vi "Re-write README files.vi"() -> ()   [LabVIEW 2010]
uses:
  <vilib>/Utility/file.llb/Read From Spreadsheet File (string).vi
  <vilib>/Utility/file.llb/Write To Spreadsheet File (string).vi
panel:
  in  "System Save Button":bool
  in  "Primary Path":path
  out "Selected Paths":path[](array[path])
  in  "Readme Files":i32(listbox)
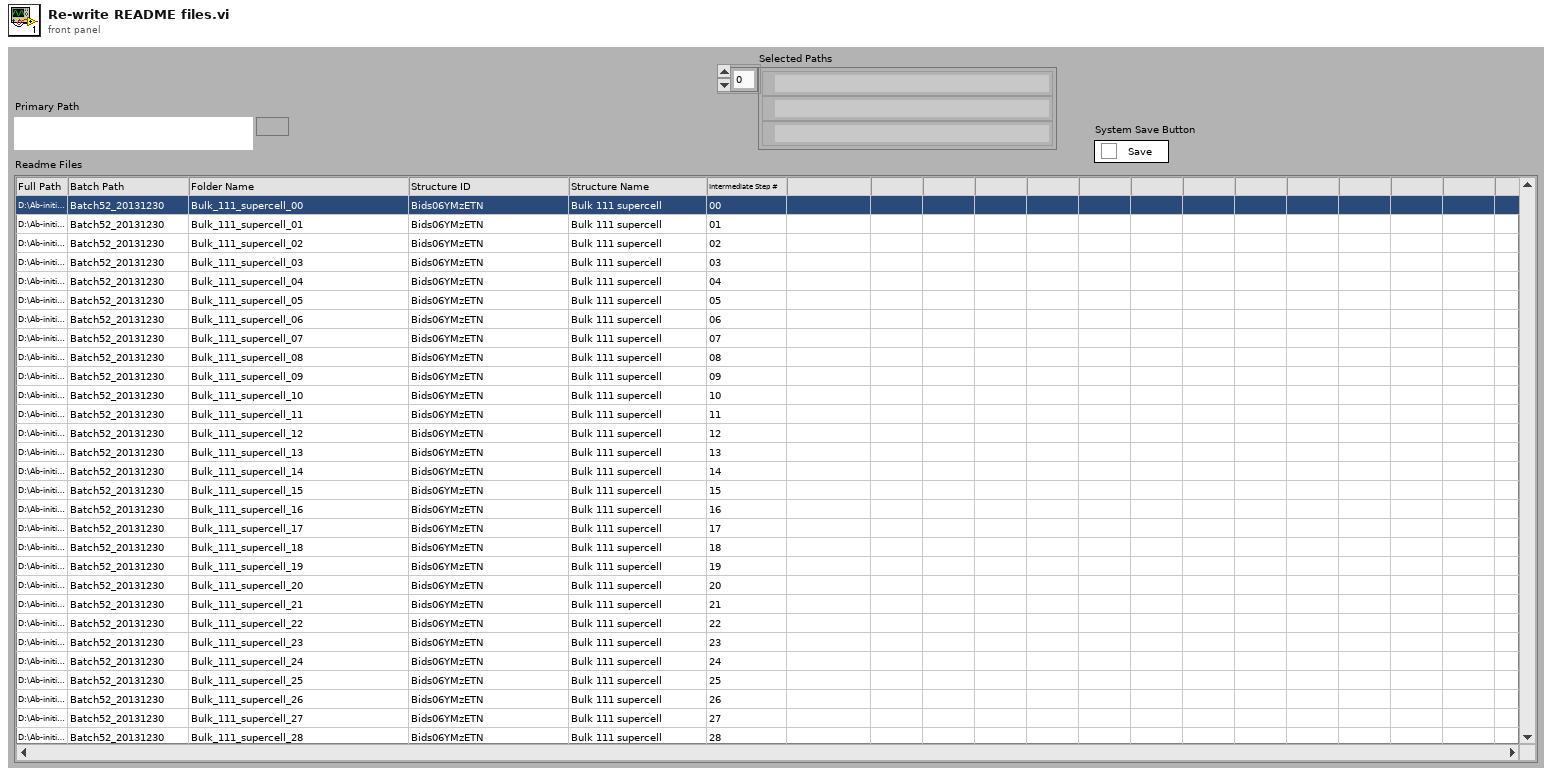
[diagram p1: front panel]
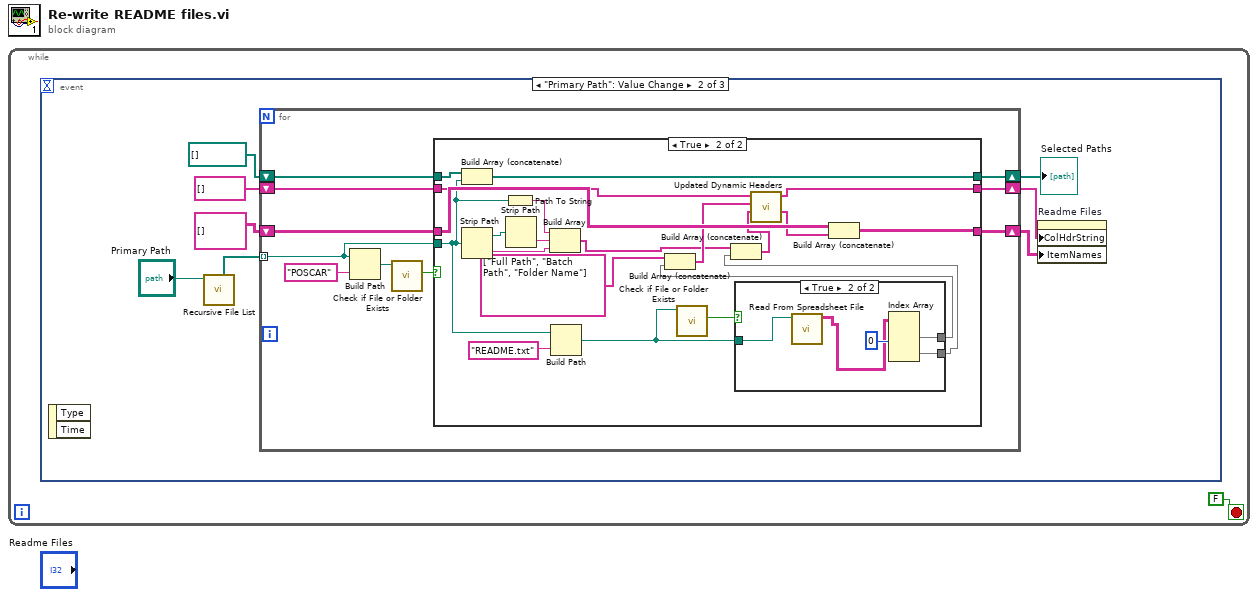
[diagram p0: block diagram]
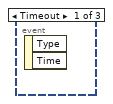
[diagram p2: hidden frame]
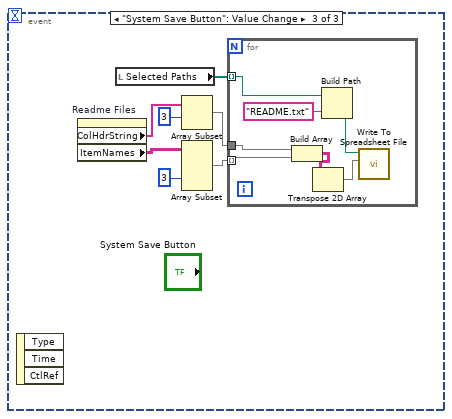
[diagram p5: hidden frame]
diagram:
  n1 = while {
    stop <- FALSE stop-if-true
    n2 = event shown="[1] \"Primary Path\": Value Change" {
      selector: _ -> [_ _ _]
      dyn-events: _ -> [_ _ _]
      timeout: _ -> [_ _ _]
      event Timeout {
        n3 = event-data() -> ()  [unwired: 1 in, 2 out]
      }
      event "Primary Path": Value Change {
        n4 = event-data() -> ()  [unwired: 1 in, 2 out]
        n5 = call <vilib>:"Recursive File List.vi"("Folder Path"="Primary Path") -> ("All Folders"=w3:path[])  [unwired: 6 in, 4 out]
        n6 = for {
          tunnel: w3 -> [w16] mode=indexing
          shift-right: [w15] -> w8
          shift-left: path[] [] -> [w14]
          shift-right: [w13] -> w7
          shift-left: string[][] [] -> [w12]
          shift-right: [w10] -> w6
          shift-left: string[] [] ("Merged Headers") -> [w11]
          n7 = Build Path(base path=w16, name or relative path="POSCAR") -> (appended path=w18:path)
          n8 = call <vilib>:"Check if File or Folder Exists.vi"("path"=w18) -> ("file or folder exists?"=w17:bool)  [unwired: 8 in, 2 out]
          n9 = case shown="True" w17 {
            tunnel: w16 -> [_ w34]
            tunnel: [w22 w43] -> w15
            tunnel: w14 -> [w22 w42]
            tunnel: [w21 w23] -> w13
            tunnel: w12 -> [w21 w37]
            tunnel: w11 -> [w20 w32]
            tunnel: [w20 w31] -> w10
            frame False {
            }
            frame True {
              n10 = Build Array (concatenate)(w42, w34) -> (w43:path[])
              n11 = Strip Path(path=w34) -> (stripped path=w40:path, name=w39:string)
              n12 = Path To String(path=w34) -> (string=w41:string)
              n13 = Strip Path(path=w40) -> (name=w38:string)  [unwired: 1 out]
              n14 = Build Array(w41, w38, w39) -> (w27:string[])
              n15 = Build Path(base path=w34, name or relative path="README.txt") -> (appended path=w36:path)
              n16 = call <vilib>:"Check if File or Folder Exists.vi"("path"=w36) -> ("file or folder exists?"=w35:bool)  [unwired: 8 in, 2 out]
              n17 = case shown="True" w35 {
                tunnel: w36 -> [_ w48]
                tunnel: [_ w46] -> w29
                tunnel: [_ w45] -> w26
                frame False {
                }
                frame True {
                  n18 = call-poly <vilib>:"Read From Spreadsheet File.vi"("file path (dialog if empty)"=w48) -> ("all rows"=w44:string[][])  [unwired: 6 in, 4 out]
                  n19 = Index Array(array=w44, index (col) #1=0 ("disabled index (col)")) -> (element #1=w46:string[], element #2=w45:string[])  [unwired: 3 in]
                }
              }
              n20 = Build Array (concatenate)(string[] ["Full Path", "Batch Path", "Folder Name"], w29) -> (w28:string[])
              n21 = Build Array (concatenate)(w27, w26) -> (w25:string[])
              n22 = call "Updated Dynamic Headers.vi"("New Data"=w25, "This Data's Headers"=w28, "Old Headers"=w32) -> ("Formatted New Data"=w24:string[], "Merged Headers"=w31:string[])  [unwired: 7 in]
              n23 = Build Array (concatenate)(w37, w24) -> (w23:string[][])
            }
          }
        }
        "Selected Paths" <- w8
        n24 = property on="Readme Files" class="MCListbox (strict)"("ColHdrString"=w6, "ItemNames"=w7) -> ()  [unwired: 2 in, 2 out]
      }
      event "System Save Button": Value Change {
        n25 = event-data() -> ()  [unwired: 1 in, 3 out]
        n26 = property on="Readme Files" class="MCListbox (strict)"() -> ("ColHdrString"=w54:string[], "ItemNames"=w51:string[][])  [unwired: 2 in, 2 out]
        n27 = local read "Selected Paths"() -> (w55:path[])
        n28 = Array Subset(array=w54, index=3) -> (w52:string[])  [unwired: 1 in]
        n29 = Array Subset(array=w51, index (col)=3 ("index")) -> (w50:string[][])  [unwired: 3 in]
        n30 = for {
          tunnel: w55 -> [w60] mode=indexing
          tunnel: w50 -> [w61] mode=indexing
          tunnel: w52 -> [w62]
          n31 = Build Array(w62, w61) -> (w57:string[][])
          n32 = Transpose 2D Array(2D array=w57) -> (transposed array=w56:string[][])
          n33 = Build Path(base path=w60, name or relative path="README.txt") -> (appended path=w58:path)
          n34 = call-poly <vilib>:"Write To Spreadsheet File.vi"("2D data"=w56, "file path (dialog if empty)"=w58) -> ()  [unwired: 6 in, 1 out]
        }
      }
    }
  }
